vi "mqttCmdAcknowledge.vi"(0 "_mqtt in":refnum<class "PublishMqttMsg.lvclass">, 11 "error in (no error)":errorcluster) -> (4 "_mqtt out":refnum<class "PublishMqttMsg.lvclass">, 8 "notification":T1, 15 "error out":errorcluster)   [LabVIEW 2020]
uses:
  mqttTypedef/mqttMessageType.ctl
  MQTT Client.lvclass
  mqttTypedef/mqttQOSlevel.ctl
  mqttTypedef/mqttFixedHeaderResponse.ctl
  mqttTypedef/mqttRXdataCluster.ctl
  PublishMqttMsg.lvclass
  C:/Projects/Libraries/Gore SM 2020/mqtt-LabVIEW/src/class/mqtt/mqttCmd/BaseMqttMsg.lvclass
  C:/Projects/Libraries/Gore SM 2020/mqtt-LabVIEW/src/class/mqtt/mqttCmd/mqttCmdPublish/PublishMqttMsg.lvclass
panel:
  out "timed out? 2":bool
  out "timed out?":bool
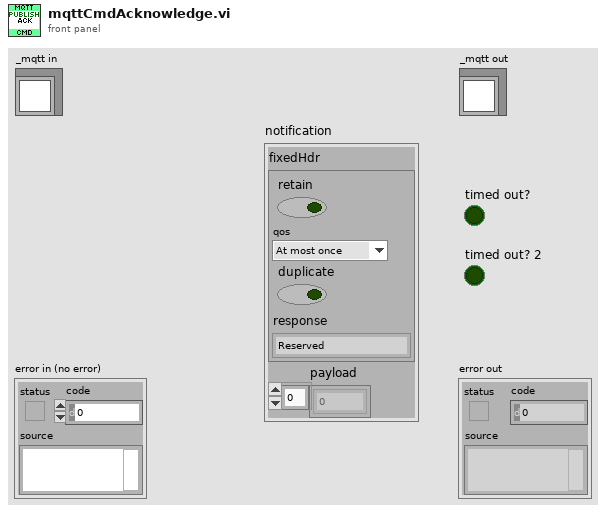
[diagram p1: front panel]
types:
  T1 = typedef "MQTT Client.lvclass/mqttRXdataCluster.ctl" = cluster{"fixedHdr":T2, "payload":u8[]}
  T2 = typedef "MQTT Client.lvclass/mqttFixedHeaderResponse.ctl" = cluster{"retain":bool, "qos":T3, "duplicate":bool, "response":T4}
  T3 = typedef "MQTT Client.lvclass/mqttQOSlevel.ctl" = enum8{"At most once", "At least once", "Exactly once", "Reserved"}
  T4 = typedef "MQTT Client.lvclass/mqttMessageType.ctl" = enum32{"Reserved", "CONNECT", "CONNACK", "PUBLISH", "PUBACK", "PUBREC", "PUBREL", "PUBCOMP", "SUBSCRIBE", "SUBACK", "UNSUBSCRIBE", "UNSUBACK", "PINGREQ", "PINGRESP", "DISCONNECT", "Reserved2"}
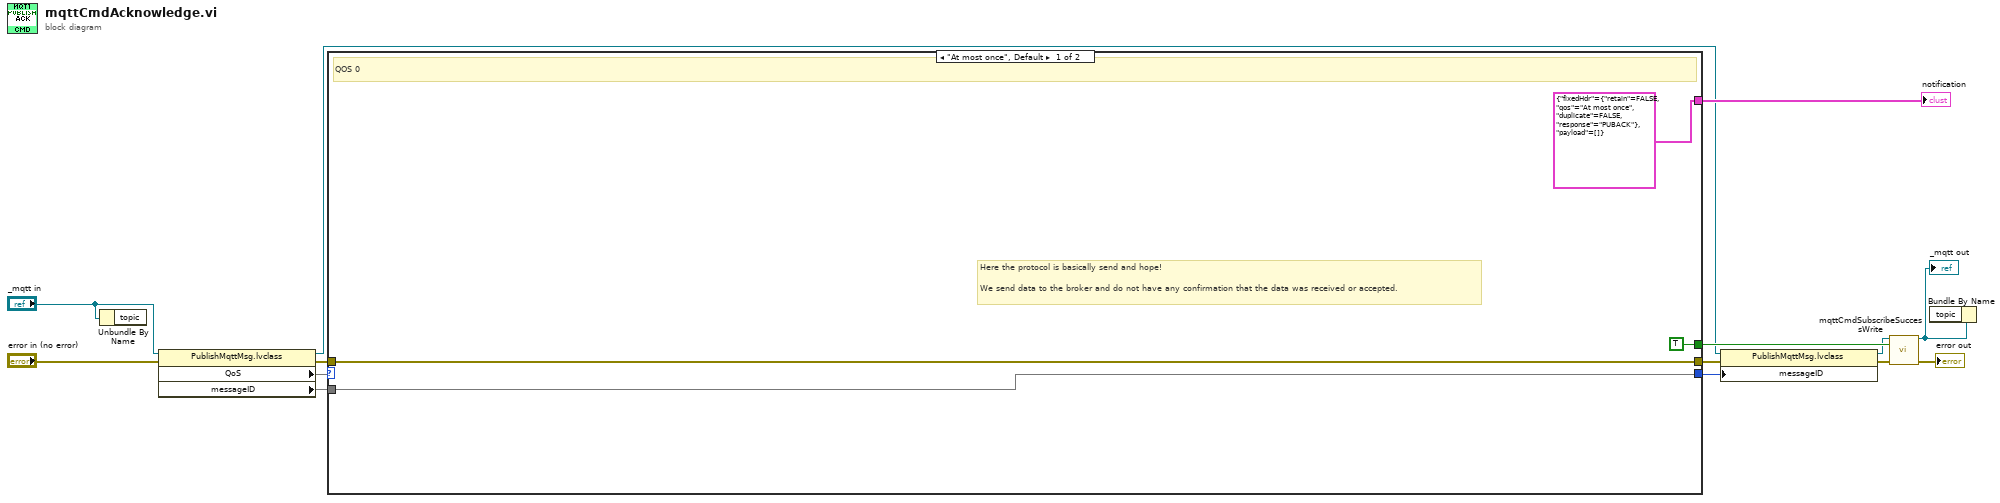
[diagram p0: block diagram]
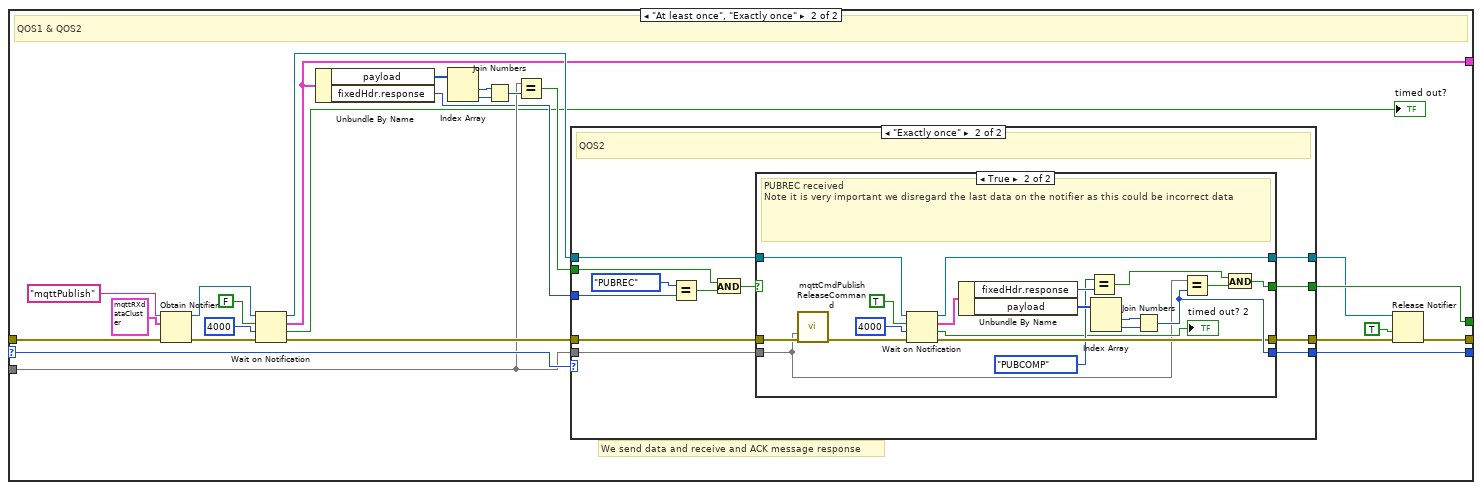
[diagram p2: hidden frame]
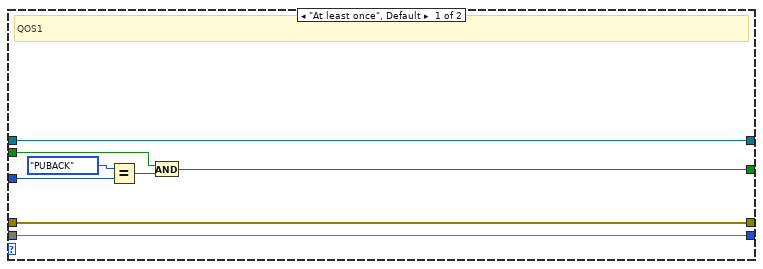
[diagram p3: hidden frame]
diagram:
  n1 = Unbundle By Name("_mqtt in") -> ()  [unwired: 1 out]
  n2 = property class="PublishMqttMsg.lvclass"(reference="_mqtt in", error in="error in (no error)") -> (reference out=w4:refnum<class "PublishMqttMsg.lvclass">, error out=w8:errorcluster, "QoS"=w6, "messageID"=w7)
  n3 = case shown="\"At most once\", Default" w6 {
    selector: w6 -> [_ w43]
    tunnel: [w18 w30] -> w5
    tunnel: w8 -> [w18 w37]
    tunnel: [w15 w41] -> w3
    tunnel: [TRUE w42] -> w11
    tunnel: w7 -> [w15 w24]
    tunnel: [T1 {"fixedHdr"={"retain"=FALSE, "qos"=enum."At most once", "duplicate"=FALSE, "response"=enum."PUBACK"}, "payload"=[]} ("notification") w21] -> w13
    frame "At most once", Default {
      # "Here the protocol is basically send and hope!\n\nWe send data to the broker and do not have any confirmation that the data was received or accepted."
      # "QOS 0"
    }
    frame "At least once", "Exactly once" {
      # "We send data and receive and ACK message response"
      # "QOS1 & QOS2"
      n4 = Obtain Notifier(name (unnamed)="mqttPublish", notification data type=T1 {"fixedHdr"={"retain"=FALSE, "qos"=enum."At most once", "duplicate"=FALSE, "response"=enum."Reserved"}, "payload"=[]} ("notification"), error in (no error)=w37) -> (notifier out=w35:refnum<notifier>, error out=w40:errorcluster)  [unwired: 1 in, 1 out]
      n5 = Wait on Notification(notifier=w35, ignore previous (F)=FALSE, timeout in ms (-1)=4000, error in (no error)=w40) -> (notifier out=w34:refnum<notifier>, notification=w21:T1, timed out?=→"timed out?":bool, error out=w36:errorcluster)
      n6 = Unbundle By Name(w21) -> ("payload"=w26:u8[], "fixedHdr.response"=w22:T4)
      n7 = Index Array(array=w26) -> (element #1=w27:u8, element #2=w28:u8)  [unwired: 2 in]
      n8 = Join Numbers(hi=w27, lo=w28) -> ((hi.lo)=w25:u16)
      n9 = Equal?(x=w24, y=w25) -> (x = y?=w23:bool)
      n10 = case shown="\"Exactly once\"" w43 {
        tunnel: [w44 w61] -> w42
        tunnel: [w51 w63] -> w32
        tunnel: w36 -> [w51 w62]
        tunnel: w24 -> [w47 w53]
        tunnel: [w47 w60] -> w41
        tunnel: w22 -> [w49 w58]
        tunnel: w34 -> [w48 w57]
        tunnel: [w48 w54] -> w33
        tunnel: w23 -> [w46 w52]
        frame "At least once", Default {
          # "QOS1"
          n11 = Equal?(x=mqttMessageType."PUBACK", y=w49) -> (x = y?=w45:bool)
          n12 = And(x=w46, y=w45) -> (x .and. y?=w44:bool)
        }
        frame "Exactly once" {
          # "QOS2"
          n13 = Equal?(x=mqttMessageType."PUBREC", y=w58) -> (x = y?=w56:bool)
          n14 = And(x=w52, y=w56) -> (x .and. y?=w55:bool)
          n15 = case shown="True" w55 {
            selector: w55 -> [w67 _]
            tunnel: [w66 w83] -> w63
            tunnel: w62 -> [w66 w70]
            tunnel: [w67 w86] -> w61
            tunnel: w53 -> [w65 w69]
            tunnel: [w65 w85] -> w60
            tunnel: w57 -> [w64 w84]
            tunnel: [w64 w82] -> w54
            frame False {
            }
            frame True {
              # "PUBREC received\nNote it is very important we disregard the last data on the notifier as this could be incorrect data"
              n16 = call "mqttCmdPublishReleaseCommand.vi"("messageID"=w69, "error in (no error)"=w70) -> ("error out"=w68:errorcluster)  [unwired: 13 in]
              n17 = Wait on Notification(notifier=w84, ignore previous (F)=TRUE, timeout in ms (-1)=4000, error in (no error)=w68) -> (notifier out=w82:refnum<notifier>, notification=w78:T1, timed out?=→"timed out? 2":bool, error out=w83:errorcluster)
              n18 = Unbundle By Name(w78) -> ("fixedHdr.response"=w76:T4, "payload"=w77:u8[])
              n19 = Equal?(x=mqttMessageType."PUBCOMP", y=w76) -> (x = y?=w74:bool)
              n20 = Index Array(array=w77) -> (element #1=w80:u8, element #2=w81:u8)  [unwired: 2 in]
              n21 = Join Numbers(hi=w80, lo=w81) -> ((hi.lo)=w85:u16)
              n22 = Equal?(x=w69, y=w85) -> (x = y?=w73:bool)
              n23 = And(x=w74, y=w73) -> (x .and. y?=w86:bool)
            }
          }
        }
      }
      n24 = Release Notifier(notifier=w33, force destroy? (F)=TRUE, error in (no error)=w32) -> (error out=w30:errorcluster)  [unwired: 2 out]
    }
  }
  "notification" <- w13
  n25 = property class="PublishMqttMsg.lvclass"(reference=w4, error in=w5, "messageID"=w3) -> (reference out=w2:refnum<class "PublishMqttMsg.lvclass">, error out=w1:errorcluster)
  n26 = call "mqttCmdSubscribeSuccessWrite.vi"("mqttBrokerCommand in"=w2, "success"=w11, "error in (no error)"=w1) -> ("mqttBrokerCommand out"=w9:refnum<class "mqttCmdPublish.lvclass">, "error out"=→"error out":errorcluster)  [unwired: 11 in]
  "_mqtt out" <- w9
  n27 = Bundle By Name(cluster=w9) -> ()  [unwired: 1 in, 1 out]
